vi "Wait (us).vi"(7 "micorseconds to wait":u64 format="%#.7p", 11 "error in (no error)":errorcluster) -> (15 "error out":errorcluster)   [LabVIEW 2011]
doc: "Yeilds the thread for the specified number of microseconds before returning.\n\nWindows Server 2003 and later: A value of zero causes the thread to relinquish the remainder of its time slice to any other thread that is ready to run. If there are no other threads ready to run, the function returns immediately, and the thread continues execution.\n\nWindows XP/2000: A value of zero causes the thread to relinquish the remainder of its time slice to any other thread of equal priority that is ready to run. If there are no other threads of equal priority ready to run, the function returns immediately, and the thread continues execution."
uses:
  kernel32.dll
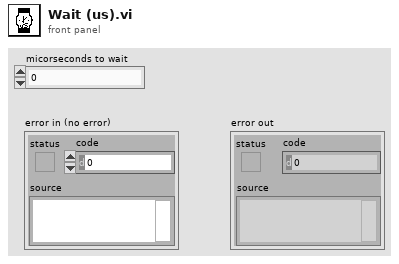
[diagram p1: front panel]
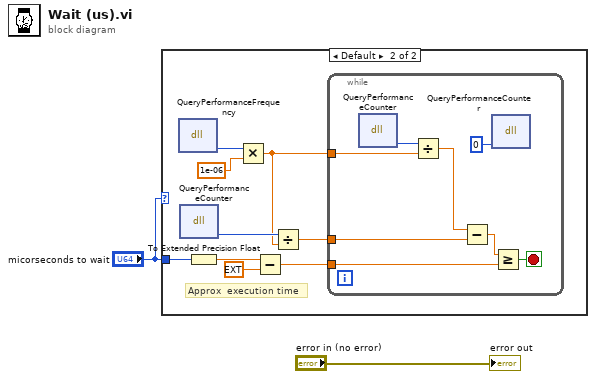
[diagram p0: block diagram]
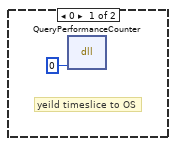
[diagram p2: hidden frame]
diagram:
  n1 = case shown="Default" "micorseconds to wait" {
    tunnel: "micorseconds to wait" -> [_ w11]
    frame 0 {
      # "yeild timeslice to OS"
      n2 = dll-call lib="kernel32.dll" fn="QueryPerformanceCounter"("dwMilliseconds"=u32 0) -> ()  [unwired: 5 in, 2 out]
    }
    frame Default {
      # "Approx  execution time"
      n3 = dll-call lib="kernel32.dll" fn="QueryPerformanceFrequency"() -> ("pTicksPerSecond"=w10:u64)  [unwired: 5 in, 2 out]
      n4 = dll-call lib="kernel32.dll" fn="QueryPerformanceCounter"() -> ("pPerformanceCount"=w12:u64)  [unwired: 5 in, 2 out]
      n5 = To Extended Precision Float(1:w11) -> (0:w6:ext)
      n6 = Multiply(x=w10, y=1e-06) -> (x*y=w7:dbl)
      n7 = Subtract(x=w6, y=ext 7.0) -> (x-y=w5:ext)
      n8 = Divide(x=w12, y=w7) -> (x/y=w8:dbl)
      n9 = while {
        tunnel: w5 -> [w16]
        tunnel: w7 -> [w18]
        tunnel: w8 -> [w19]
        stop <- w14 stop-if-true
        n10 = dll-call lib="kernel32.dll" fn="QueryPerformanceCounter"() -> ("pPerformanceCount"=w20:u64)  [unwired: 5 in, 2 out]
        n11 = Divide(x=w20, y=w18) -> (x/y=w17:dbl)
        n12 = Subtract(x=w17, y=w19) -> (x-y=w15:dbl)
        n13 = dll-call lib="kernel32.dll" fn="QueryPerformanceCounter"("dwMilliseconds"=u32 0) -> ()  [unwired: 5 in, 2 out]
        n14 = Greater Or Equal?(x=w15, y=w16) -> (x >= y?=w14:bool)
      }
    }
  }
  "error out" <- "error in (no error)"
